vi "controllerMain.vi"(8 "error in (no error)":errorcluster, 10 "UserEvents in":refnum<class "UserEvents.lvclass">, 11 "Controller in":refnum<class "Controller.lvclass">) -> (0 "error out":errorcluster, 3 "Controller out":refnum<class "Controller.lvclass">)   [LabVIEW 2013, in "Controller.lvclass"]
uses:
  Controller.lvclass
  StateFactory/StateFactory.lvclass
  Typedefs/StateSelector.ctl
  Typedefs/M2AADTTypedefs.lvlib
  Model/Model/Model.lvclass
  Command/Command.lvclass
  Context/Context.lvclass
  CommandFactory/CommandFactory.lvclass
  UserEvents/UserEvents.lvclass
  <userlib>/Common/SerialProtocols/SerialProtocolFactory/SerialProtocolFactory/SerialProtocolFactory.lvclass
  <userlib>/Common/SerialProtocols/SerialCommunicator/SerialCommunicator.lvclass
  <userlib>/Common/ILC/ILC/ILC.lvclass
  <userlib>/Common/Devices/DistanceGauge/DistanceGauge/DistanceGauge.lvclass
  <userlib>/Common/Simulators/DistanceGaugeSim/DistanceGaugeSim.lvclass
  Model/ApplicationElements/SystemController/SystemController.lvclass
  Model/ApplicationElements/TestMonitor/TestMonitor.lvclass
  Model/ApplicationElements/ApplicationElements.ctl
  Model/ApplicationElements/StiffnessMonitor/StiffnessMonitor.lvclass
  Model/ApplicationElements/Thermocouple/Thermocouple.lvclass
  Model/ApplicationElements/Log/TestDataLog/TestDataLog.lvclass
  Model/ApplicationElements/Log/StiffnessLog/StiffnessLog.lvclass
  Model/ILCTC/ILCTC.lvclass
  Model/ApplicationElements/DistanceGaugeTC/DistanceGaugeTC.lvclass
  Model/ApplicationElements/StepperMotorTC/StepperMotorTC.lvclass
  Model/ApplicationElements/ForceSensorCalculatorTC/ForceSensorCalculatorTC.lvclass
  Model/ApplicationElements/EncoderConverterTC/EncoderConverterTC.lvclass
  Model/ILCSim1TC/ILCSim1TC.lvclass
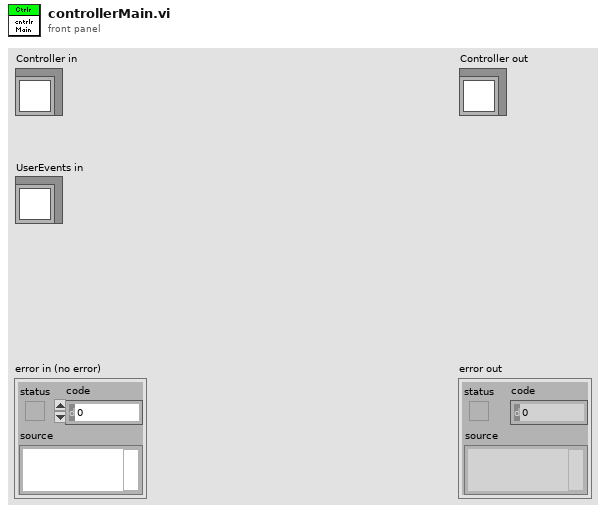
[diagram p1: front panel]
types:
  T1 = typedef "ApplicationElements.ctl" = cluster{"distanceGaugeTC":refnum<class "DistanceGaugeTC.lvclass">, "forceSensorCalculatorTC":refnum<class "ForceSensorCalculatorTC.lvclass">, "systemController":refnum<class "SystemController.lvclass">, "stepperMotorTC":refnum<class "StepperMotorTC.lvclass">, "testMonitor":refnum<class "TestMonitor.lvclass">, "testDataLog":refnum<class "TestDataLog.lvclass">, "stiffnessLog":refnum<class "StiffnessLog.lvclass">, "encoderConverterTC":refnum<class "EncoderConverterTC.lvclass">, "stiffnessMonitor":refnum<class "StiffnessMonitor.lvclass">, "thermocouple":refnum<class "Thermocouple.lvclass">}
  T2 = typedef "M2AADTTypedefs.lvlib/StateSelector.ctl" = enum16{"EndingCycleState", "FaultState", "InteractiveMotionState", "MovingToNewForceState", "OffState", "PausingState", "StandbyState", "StoppedState"}
  T3 = typedef "M2AADTTypedefs.lvlib/SubDataEvents.ctl" = cluster{"Command":refnum<user-event>}
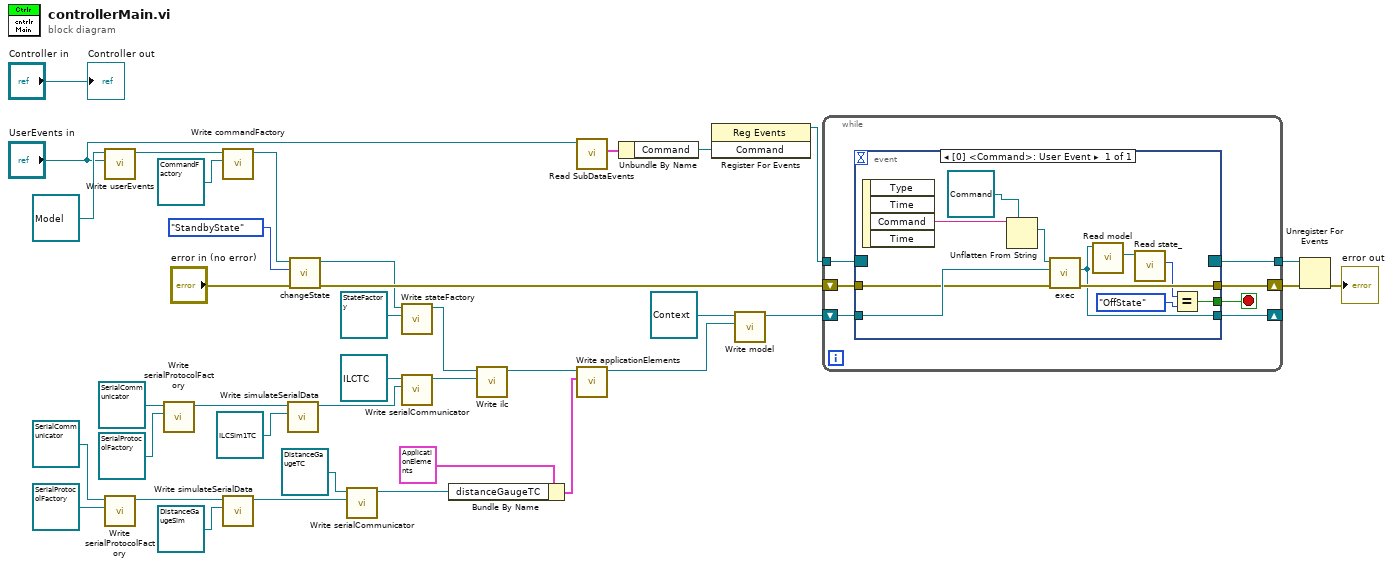
[diagram p0: block diagram]
diagram:
  n1 = call "Write userEvents.vi"("userEvents"="UserEvents in", "Model in"=refnum<class "Model.lvclass"> refnum) -> ("Model out"=w9:refnum<class "Model.lvclass">)  [unwired: 9 in]
  n2 = call <userlib>:"Write serialProtocolFactory.vi"("serialProtocolFactory"=refnum<class "SerialProtocolFactory.lvclass"> refnum ("SerialCommFactory.lvclass"), "SerialCommunicator in"=refnum<class "SerialCommunicator.lvclass"> refnum ("SerialProtocols.lvlib:SerialCommunicator.lvclass")) -> ("SerialCommunicator out"=w4:refnum<class "SerialCommunicator.lvclass">)  [unwired: 9 in]
  n3 = call <userlib>:"Write serialProtocolFactory.vi"("serialProtocolFactory"=refnum<class "SerialProtocolFactory.lvclass"> refnum ("SerialCommFactory.lvclass"), "SerialCommunicator in"=refnum<class "SerialCommunicator.lvclass"> refnum ("SerialProtocols.lvlib:SerialCommunicator.lvclass")) -> ("SerialCommunicator out"=w22:refnum<class "SerialCommunicator.lvclass">)  [unwired: 9 in]
  n4 = call "Write commandFactory.vi"("commandFactory"=refnum<class "CommandFactory.lvclass"> refnum ("CommandFactory.lvclass"), "Model in"=w9) -> ("Model out"=w7:refnum<class "Model.lvclass">)  [unwired: 9 in]
  n5 = call <userlib>:"Write simulateSerialData.vi"("simulateSerialData"=refnum<class "DistanceGaugeSim.lvclass"> refnum ("DistanceGaugeSim.lvclass"), "SerialCommunicator in"=w4) -> ("SerialCommunicator out"=w17:refnum<class "SerialCommunicator.lvclass">)  [unwired: 9 in]
  n6 = call <userlib>:"Write simulateSerialData.vi"("simulateSerialData"=refnum<class "ILCSim1TC.lvclass"> refnum ("ILCSim1TC.lvclass"), "SerialCommunicator in"=w22) -> ("SerialCommunicator out"=w21:refnum<class "SerialCommunicator.lvclass">)  [unwired: 9 in]
  n7 = call "changeState.vi"("error in (no error)"="error in (no error)", "State:"=StateSelector."StandbyState", "Model in"=w7) -> ("error out"=w29:errorcluster, "Model out"=w5:refnum<class "Model.lvclass">)  [unwired: 7 in]
  n8 = call <userlib>:"Write serialCommunicator.vi"("serialCommunicator"=w17, "DistanceGauge in"=refnum<class "DistanceGaugeTC.lvclass"> refnum ("DistanceGaugeTC.lvclass")) -> ("DistanceGauge out"=w13:refnum<class "DistanceGaugeTC.lvclass">)  [unwired: 9 in]
  n9 = call "Write stateFactory.vi"("stateFactory"=refnum<class "StateFactory.lvclass"> refnum ("StateFactory.lvclass"), "Model in"=w5) -> ("Model out"=w23:refnum<class "Model.lvclass">)  [unwired: 9 in]
  n10 = call <userlib>:"Write serialCommunicator.vi"("serialCommunicator"=w21, "ILC in"=refnum<class "ILCTC.lvclass"> refnum ("ILC_TC.lvclass")) -> ("ILC out"=w24:refnum<class "ILCTC.lvclass">)  [unwired: 9 in]
  n11 = Bundle By Name(cluster=T1 {"distanceGaugeTC"=refnum, "forceSensorCalculatorTC"=refnum, "systemController"=refnum, "stepperMotorTC"=refnum, "testMonitor"=refnum, "testDataLog"=refnum, "stiffnessLog"=refnum, "encoderConverterTC"=refnum, "stiffnessMonitor"=refnum, "thermocouple"=refnum} ("applicationElements"), "distanceGaugeTC"=w13) -> (w12:T1)
  n12 = call "Write ilc.vi"("ilc"=w24, "Model in"=w23) -> ("Model out"=w16:refnum<class "Model.lvclass">)  [unwired: 9 in]
  n13 = call "Read SubDataEvents.vi"("UserEvents in"="UserEvents in") -> ("SubDataEvents"=w33:T3)  [unwired: 9 in, 1 out]
  n14 = call "Write applicationElements.vi"("applicationElements"=w12, "Model in"=w16) -> ("Model out"=w15:refnum<class "Model.lvclass">)  [unwired: 9 in]
  n15 = Unbundle By Name(w33) -> ("Command"=w27:refnum<user-event>)
  n16 = register-events(w27) -> (reference out=w32:refnum<event-registration>)  [unwired: 2 in, 1 out]
  n17 = call "Write model.vi"("Model.lvclass"=w15, "Context in"=refnum<class "Context.lvclass"> refnum ("Context.lvclass")) -> ("Context out"=w35:refnum<class "Context.lvclass">)  [unwired: 9 in]
  n18 = while {
    shift-right: [w44] -> w30
    shift-left: w29 -> [w41]
    shift-right: [w43] -> _
    shift-left: w35 -> [w45]
    tunnel: w32 -> [w40]
    tunnel: [w39] -> w31
    stop <- w42 stop-if-true
    n19 = event shown="[0] <Command>: User Event" {
      selector: w40 -> [_]
      dyn-events: [_] -> w39
      timeout: _ -> [_]
      tunnel: w45 -> [w54]
      tunnel: [w51] -> w44
      tunnel: [w50] -> w43
      tunnel: [w49] -> w42
      tunnel: w41 -> [w47]
      event User Event {
        n20 = event-data() -> ("Command"=w46:string)  [unwired: 1 in, 3 out]
        n21 = Unflatten From String(type=refnum<class "Command.lvclass"> refnum ("Command.lvclass"), binary string=w46) -> (value=w55:refnum<class "Command.lvclass">)  [unwired: 3 in, 2 out]
        n22 = call-dynamic "exec.vi"("error in (no error)"=w47, "context"=w54, "Command in"=w55) -> ("error out"=w51:errorcluster, "context 2"=w50:refnum<class "Context.lvclass">)  [unwired: 6 in, 1 out]
        n23 = call "Read model.vi"("Context in"=w50) -> ("Model.lvclass"=w53:refnum<class "Model.lvclass">)  [unwired: 9 in, 1 out]
        n24 = call "Read state_.vi"("Model in"=w53) -> ("state:"=w48:T2)  [unwired: 9 in, 1 out]
        n25 = Equal?(x=w48, y=StateSelector."OffState") -> (x = y?=w49:bool)
      }
    }
  }
  n26 = Unregister For Events(event registration refnum=w31, error in=w30) -> (error out=→"error out":errorcluster)
  "Controller out" <- "Controller in"
